vi "UE_Driver.vi"(2 "TVID_Operation_Select":T1, 11 "Error_In":errorcluster) -> (4 "Event_Registration_Refnum":refnum<event-registration>, 6 "Stop":refnum<user-event>, 15 "Error_Out":errorcluster)   [LabVIEW 2021]
doc: "Used to Create, generate and destory the User event"
uses:
  Controls/UE_Driver_Operation_Select.ctl
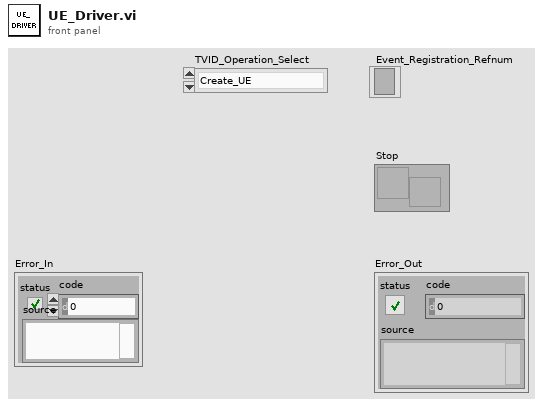
[diagram p1: front panel]
types:
  T1 = typedef "UE_Driver_Operation_Select.ctl" = enum16{"Create_UE", "Get_Refnum", "Generate_UE", "Destroy_UE"}
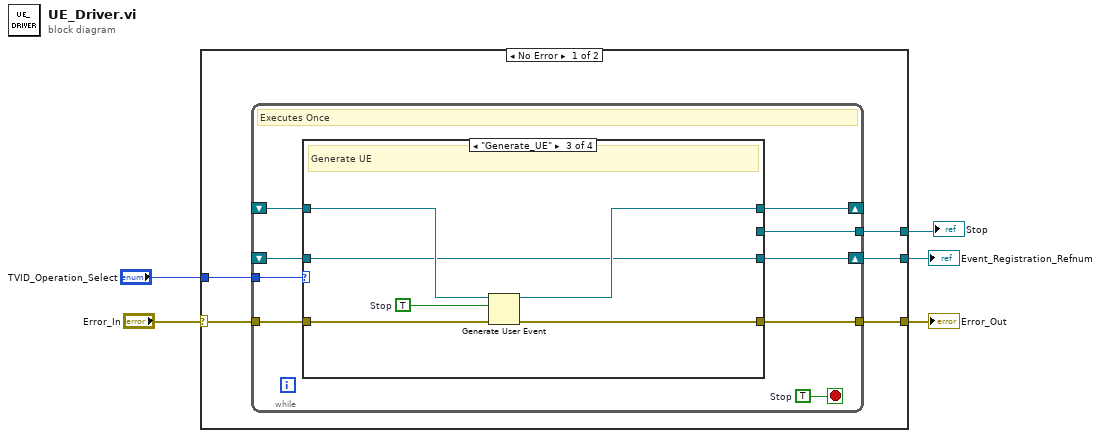
[diagram p0: block diagram]
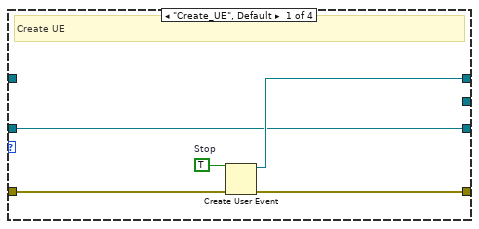
[diagram p2: hidden frame]
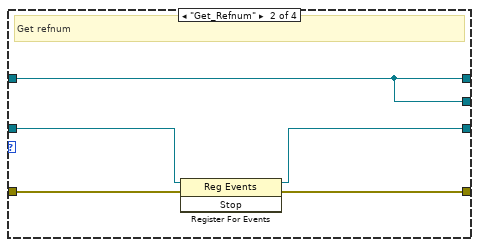
[diagram p3: hidden frame]
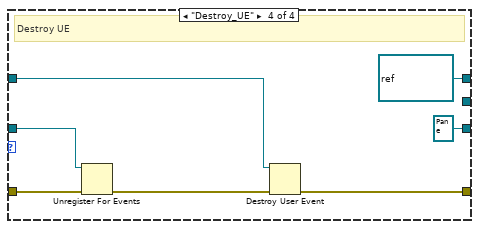
[diagram p4: hidden frame]
diagram:
  n1 = case shown="No Error" "Error_In" {
    selector: "Error_In" -> [w10 w43]
    tunnel: "TVID_Operation_Select" -> [w9 _]
    tunnel: [w8 _] -> w3
    tunnel: [w7 w43] -> w2
    tunnel: [w6 _] -> w1
    frame No Error {
      n2 = while {
        shift-right: [w17] -> _
        shift-left: _ -> [w16]
        tunnel: w10 -> [w19]
        tunnel: w9 -> [w18]
        shift-right: [w14] -> w8
        shift-left: _ -> [w13]
        tunnel: [w12] -> w7
        tunnel: [w11] -> w6
        stop <- w15 stop-if-true
        w15 = TRUE  # Stop
        # "Executes Once"
        n3 = case shown="\"Generate_UE\"" w18 {
          tunnel: w19 -> [w24 w29 w35 w42]
          tunnel: [w22 w28 w34 w38] -> w12
          tunnel: [w21 w25 w31 refnum<user-event> refnum ("Stop")] -> w17
          tunnel: w16 -> [_ w25 w33 w37]
          tunnel: [w20 w27 w30 refnum<event-registration> refnum ("event registration refnum")] -> w14
          tunnel: w13 -> [w20 w26 w30 w40]
          tunnel: [_ w25 _ _] -> w11
          frame "Create_UE", Default {
            w23 = TRUE  # Stop
            # "Create UE"
            n4 = Create User Event(user event datatype=w23, error in=w24) -> (user event=w21:refnum<user-event>, error out=w22:errorcluster)
          }
          frame "Get_Refnum" {
            # "Get refnum"
            n5 = register-events(reference=w26, error in=w29) -> (reference out=w27:refnum<event-registration>, error out=w28:errorcluster)  [unwired: 1 in]
          }
          frame "Generate_UE" {
            w32 = TRUE  # Stop
            # "Generate UE"
            n6 = Generate User Event(user event=w33, event data cluster=w32, error in=w35) -> (user event out=w31:refnum<user-event>, error out=w34:errorcluster)  [unwired: 1 in]
          }
          frame "Destroy_UE" {
            # "Destroy UE"
            n7 = Unregister For Events(event registration refnum=w40, error in=w42) -> (error out=w41:errorcluster)
            n8 = Destroy User Event(user event=w37, error in=w41) -> (error out=w38:errorcluster)
          }
        }
      }
    }
    frame Error {
    }
  }
  "Event_Registration_Refnum" <- w3
  "Error_Out" <- w2
  "Stop" <- w1
